vi "Teperature and FIeld Sweep_1022D.vi"() -> ()   [LabVIEW 2022 SP3]
uses:
  <vilib>/Analysis/baseanly.llb/Mean (DBL).vi
  <vilib>/Utility/file.llb/Write Delimited Spreadsheet (DBL).vi
  <vilib>/Analysis/NI_AALBase.lvlib
panel:
  out "Rh1 B/A v F":cluster{dbl[], dbl[]}(graph)
  in  "?":bool
  out "Temperature Status":i32(ring) items=["TemperatureUnknown"=0, "Stable"=1, "Tracking"=2, "Near"=5, "Chasing"=6, "Filling"=7, "Standby"=10, "Disabled"=13, "ImpedanceNotFunction"=14, "TempFailure"=15]
  out "Field Status":i32(ring) items=["MagnetUnknown"=0, "StablePersistent"=1, "WarmingSwitch"=2, "CoolingSwitch"=3, "StableDriven"=4, "Iterating"=5, "Charging"=6, "Discharging"=7, "CurrentError"=8, "MagnetFailure"=15]
  out "Field":dbl
  out "Temperature":dbl
  in  "Initialize":bool
  in  "System Stablization (s)":dbl=0.1 format="%#_13g"
  in  "Low Value (Oe)":dbl=-30000.0
  in  "High Value (Oe)":dbl=30000.0
  in  "Sweep Field Approach":i32(ring) items=["Linear", "NoOvershoot", "Oscillate"]
  in  "Sweep F Rate (Oe/s)":dbl=200.0 format="%#_13g"
  in  "Sweep F mode":i32(ring) items=["Persistent", "Driven"]
  in  "Set Fixed T":dbl=2.0
  in  "Fixed Temperature Approach":i32(ring)=1 items=["FastSettle", "NoOvershoot"]
  in  "FIxed T  Rate (K/min)":dbl=20.0
  out "PhaseA-F":cluster{dbl[], dbl[]}(graph)
  out "RA-F":cluster{dbl[], dbl[]}(graph)
  out "Phaseh1B-F":cluster{dbl[], dbl[]}(graph)
  out "Rh1B-F":cluster{dbl[], dbl[]}(graph)
  out "phase B 2":dbl
  in  "Phase B 2":u16(ring)=3 items=["X", "Y", "R", "Theta", "Frequency", "Noise", "Xh1", "Yh1", "Rh1", "Theta h1", "Xh2", "Yh2", "Rh2", "Theta h2"]
  out "phase A 2":dbl
  in  "Phase A 2":u16(ring)=3 items=["X", "Y", "R", "Theta", "Frequency", "Noise", "Xh1", "Yh1", "Rh1", "Theta h1", "Xh2", "Yh2", "Rh2", "Theta h2"]
  out "para1 Measurement (mV) 2":dbl=1.49013e-07
  in  "F Clear Plot A":bool
  in  "Parameter A 2":u16(ring)=2 items=["X", "Y", "R", "Theta", "Frequency", "Noise", "Xh1", "Yh1", "Rh1", "Theta h1", "Xh2", "Yh2", "Rh2", "Theta h2"]
  out "para2 Measurement (uV) 2":dbl=1.49013e-07
  in  "F Clear Plot B":bool
  in  "Parameter B 2":u16(ring)=2 items=["X", "Y", "R", "Theta", "Frequency", "Noise", "Xh1", "Yh1", "Rh1", "Theta h1", "Xh2", "Yh2", "Rh2", "Theta h2"]
  out "Field Setting":dbl format="%#_13g"
  out "Fixed Temperature":dbl
  out "Measured Field":dbl
  out "Field Status":i32(ring) items=["MagnetUnknown"=0, "StablePersistent"=1, "WarmingSwitch"=2, "CoolingSwitch"=3, "StableDriven"=4, "Iterating"=5, "Charging"=6, "Discharging"=7, "CurrentError"=8, "MagnetFailure"=15]
  out "Temperature Status":i32(ring) items=["TemperatureUnknown"=0, "Stable"=1, "Tracking"=2, "Near"=5, "Chasing"=6, "Filling"=7, "Standby"=10, "Disabled"=13, "ImpedanceNotFunction"=14, "TempFailure"=15]
  out "Measuring F":bool
  in  "Step(Oe)":i32=2000
  out "F loop run":i32
  out "Temperature Status":i32(ring) items=["TemperatureUnknown"=0, "Stable"=1, "Tracking"=2, "Near"=5, "Chasing"=6, "Filling"=7, "Standby"=10, "Disabled"=13, "ImpedanceNotFunction"=14, "TempFailure"=15]
  out "Field Status":i32(ring) items=["MagnetUnknown"=0, "StablePersistent"=1, "WarmingSwitch"=2, "CoolingSwitch"=3, "StableDriven"=4, "Iterating"=5, "Charging"=6, "Discharging"=7, "CurrentError"=8, "MagnetFailure"=15]
  out "Fixed Field":dbl
  out "Measured Temperature":dbl
  in  "Delay(T/F)":dbl=3000.0
  in  "Set FIxed F (Oe)":dbl format="%#_13g"
  in  "Fixed Field Approach":i32(ring) items=["Linear", "NoOvershoot", "Oscillate"]
  in  "FIxed F Rate (Oe/s)":dbl=100.0 format="%#_13g"
  in  "Fixed F mode":i32(ring) items=["Persistent", "Driven"]
  in  "Sweep Temperature Approach":i32(ring)=1 items=["FastSettle", "NoOvershoot"]
  in  "Sweep T  Rate (K/min)":dbl=10.0
  in  "Sweep T/F":bool
  in  "Remote":bool=TRUE
  in  "IP Address":string="169.254.170.239"
  out "Measuring T":bool
  in  "A Sine Output Amplitude (V)":sgl=0.1
  in  "path (folder + filename)":string="G:\\My Drive\\Opticool\\Measurement\\TF dependence\\TaI21_A1615_B166_267Hz_20kOhm"
  in  "LOCKIN address":refnum<visa-resource-name>="COM3"
  out "PhaseA-T":cluster{dbl[], dbl[]}(graph)
  out "RA-T":cluster{dbl[], dbl[]}(graph)
  out "Phaseh1-T":cluster{dbl[], dbl[]}(graph)
  out "Rh1B-T":cluster{dbl[], dbl[]}(graph)
  out "phase B":dbl
  in  "Phase B":u16(ring)=9 items=["X", "Y", "R", "Theta", "Frequency", "Noise", "Xh1", "Yh1", "Rh1", "Theta h1", "Xh2", "Yh2", "Rh2", "Theta h2"]
  out "phase A":dbl
  in  "Phase A":u16(ring)=3 items=["X", "Y", "R", "Theta", "Frequency", "Noise", "Xh1", "Yh1", "Rh1", "Theta h1", "Xh2", "Yh2", "Rh2", "Theta h2"]
  out "para1 Measurement (mV)":dbl=1.49013e-07
  in  "T Clear Plot A":bool
  in  "Parameter A":u16(ring)=2 items=["X", "Y", "R", "Theta", "Frequency", "Noise", "Xh1", "Yh1", "Rh1", "Theta h1", "Xh2", "Yh2", "Rh2", "Theta h2"]
  out "para2 Measurement (uV)":dbl=1.49013e-07
  in  "T Clear Plot B":bool
  in  "Parameter B":u16(ring)=8 items=["X", "Y", "R", "Theta", "Frequency", "Noise", "Xh1", "Yh1", "Rh1", "Theta h1", "Xh2", "Yh2", "Rh2", "Theta h2"]
  out "Temperature Setting":dbl format="%#_13g"
  in  "Save data or not":bool=TRUE
  in  "Step(K)":i32=10
  out "T loop run":i32
  in  "B frequency":dbl=267.7 format="%#_13g"
  in  "B Input Connection (0: Single-Ended)":u16(ring)=1 items=["Single-Ended Voltage", "Differential Voltage", "1 MOhm Current Gain", "100 MOhm Current Gain"]
  in  "B harmonic 1":u8=2
  in  "B harmonic 2":u8=3
  in  "B reference Manual Phase":dbl=-59.75
  in  "auto phase B":bool=TRUE
  in  "B Sample time (s)":dbl=0.001 min=0.001 max=100.0 step=0.001
  in  "B Sensitivity":u16(ring)=20 items=["1 nV/fA", "2 nV/fA", "5 nV/fA", "10 nV/fA", "20 nV/fA", "50 nV/fA", "100 nV/fA", "200 nV/fA", "500 nV/fA", "1 uV/pA", "2 uV/pA", "5 uV/pA", "10 uV/pA", "20 uV/pA", "50 uV/pA", "100 uV/pA", "200 uV/pA", "500 uV/pA", "1 mV/nA", "2 mV/nA", "5 mV/nA", "10 mV/nA", "20 mV/nA", "50 mV/nA", "100 mV/nA", "200 mV/nA", "500 mV/nA", "1 V/uA"]
  in  "Enable Sync Filter B (open when f<200Hz)":bool
  in  "B Time Constant":u8(ring)=9 items=["10 us", "30 us", "100 us", "300 us", "1 ms", "3 ms", "10 ms", "30 ms", "100 ms", "300 ms", "1 s", "3 s", "10 s", "30 s", "100 s", "300 s", "1 ks", "3 ks"]
  in  "B Reference Source":u8(ring) items=["External", "Internal", "Internal Sweep", "Channel-A"]
  in  "B Low Pass Filter Slope":u8(ring)=2 items=["6 dB/oct", "12 dB/oct", "18 db/oct", "24 dB/oct"]
  in  "A frequency":dbl=267.7 format="%#_13g"
  in  "A Input Connection (0: Single-Ended)":u16(ring)=1 items=["Single-Ended Voltage", "Differential Voltage", "1 MOhm Current Gain", "100 MOhm Current Gain"]
  in  "A harmonic 1":u8=2
  in  "A harmonic 2":u8=3
  in  "A reference Manual Phase":dbl=-59.75
  in  "auto phase A":bool=TRUE
  in  "A Reference Source":u8(ring)=1 items=["External", "Internal", "Internal Sweep"]
  in  "A Sample time (s)":dbl=0.001 min=0.001 max=100.0 step=0.001
  in  "A Time Constant":u8(ring)=9 items=["10 us", "30 us", "100 us", "300 us", "1 ms", "3 ms", "10 ms", "30 ms", "100 ms", "300 ms", "1 s", "3 s", "10 s", "30 s", "100 s", "300 s", "1 ks", "3 ks"]
  in  "Enable Sync Filter A (open when f<200Hz)":bool
  in  "A Sensitivity":u16(ring)=20 items=["1 nV/fA", "2 nV/fA", "5 nV/fA", "10 nV/fA", "20 nV/fA", "50 nV/fA", "100 nV/fA", "200 nV/fA", "500 nV/fA", "1 uV/pA", "2 uV/pA", "5 uV/pA", "10 uV/pA", "20 uV/pA", "50 uV/pA", "100 uV/pA", "200 uV/pA", "500 uV/pA", "1 mV/nA", "2 mV/nA", "5 mV/nA", "10 mV/nA", "20 mV/nA", "50 mV/nA", "100 mV/nA", "200 mV/nA", "500 mV/nA", "1 V/uA"]
  in  "A Low Pass Filter Slope":u8(ring)=2 items=["6 dB/oct", "12 dB/oct", "18 db/oct", "24 dB/oct"]
  in  "stabilization(S)":dbl=0.1 format="%#_13g"
  in  "High Value (K)":dbl=300.0
  in  "Low Value (K)":dbl=2.0
  in  "loop #":i32=1
  # "Statue"
  # "Lock-in Setting"
  # "Channel A"
  # "Channel B"
  # "Sweep F Mesurement"
  # "Temprature and Field Setting"
  # "Sweep T Mesurement"
  # "Sweep F"
  # "Sweep T"
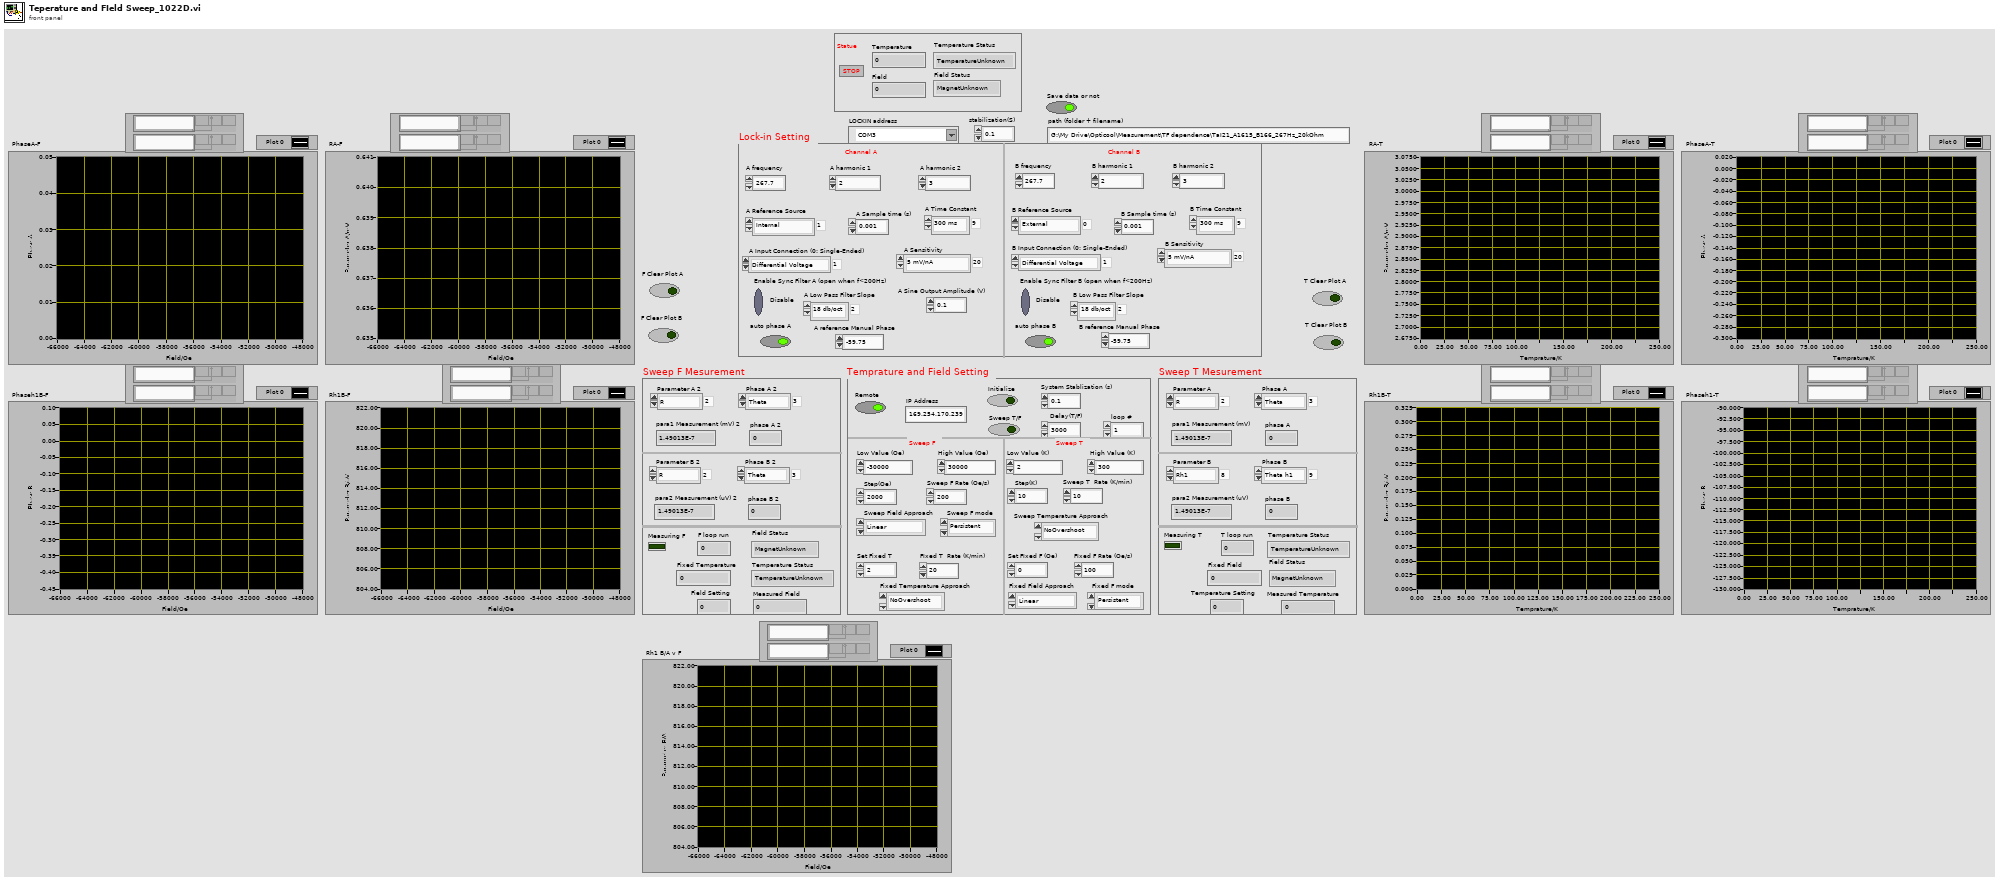
[diagram p1: front panel]
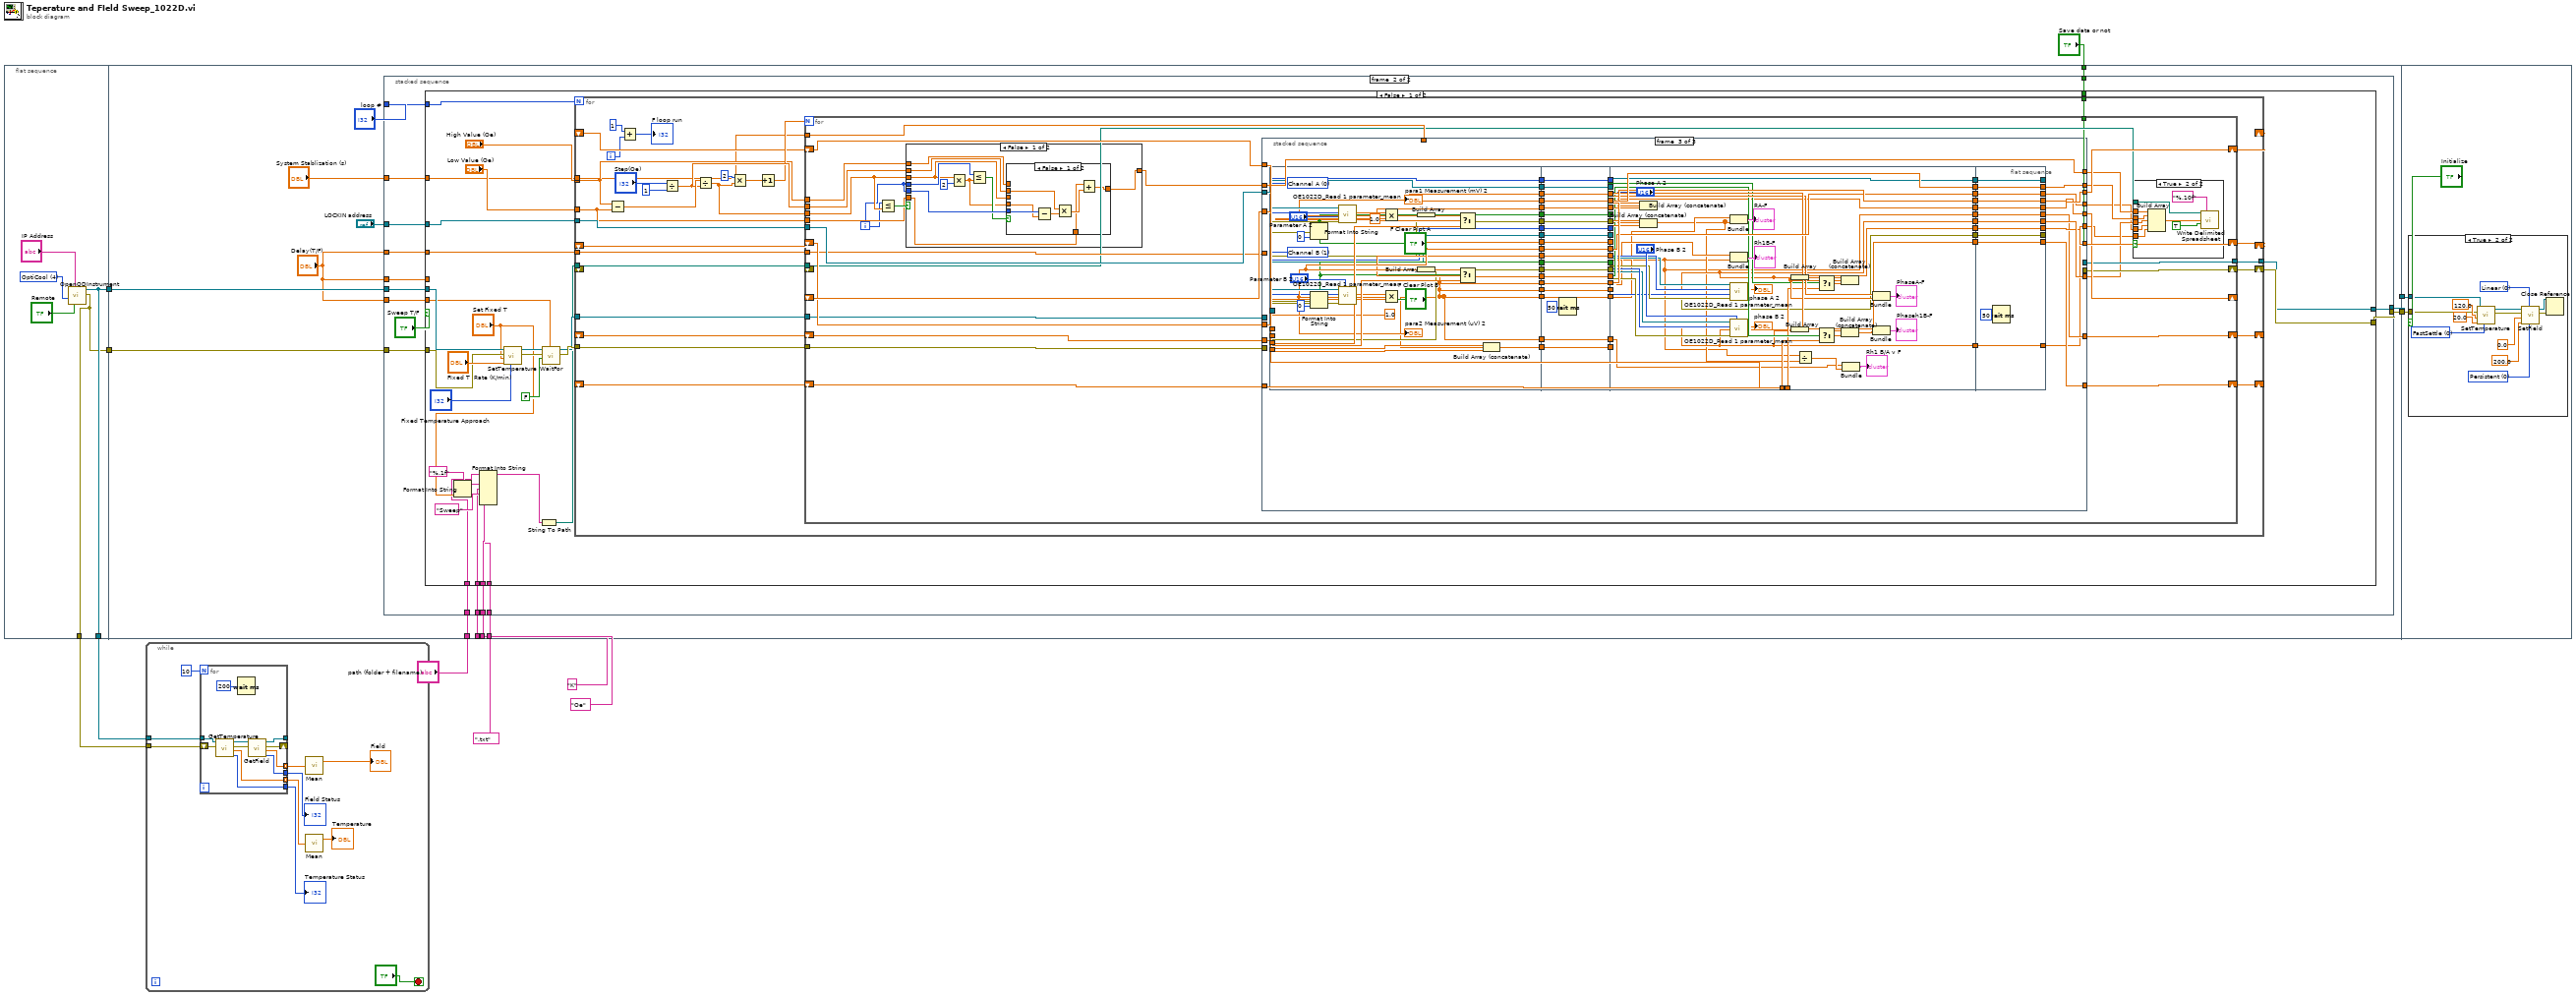
[diagram p0: block diagram]
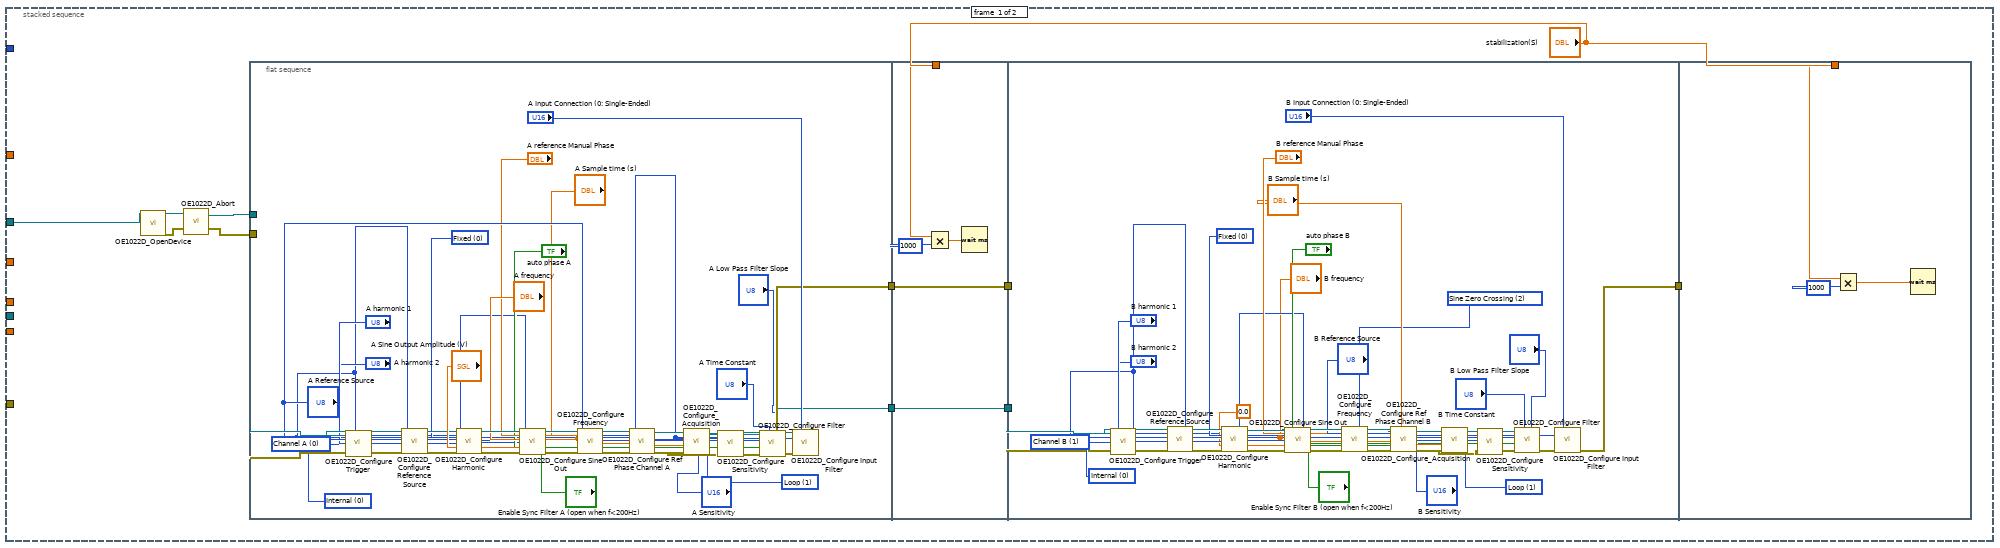
[diagram p2: hidden frame]
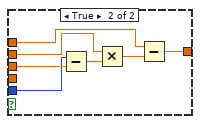
[diagram p4: hidden frame]
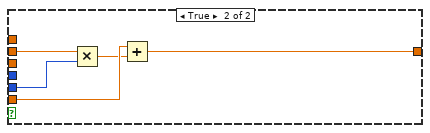
[diagram p5: hidden frame]
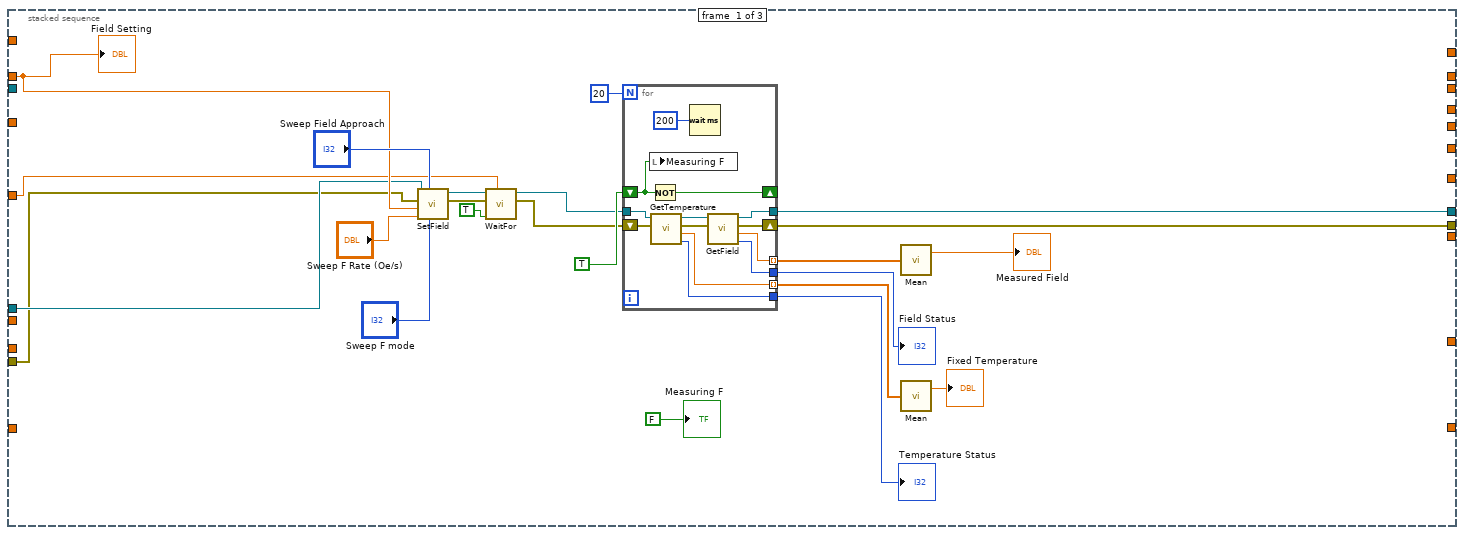
[diagram p6: hidden frame]
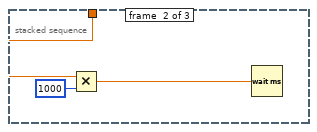
[diagram p7: hidden frame]
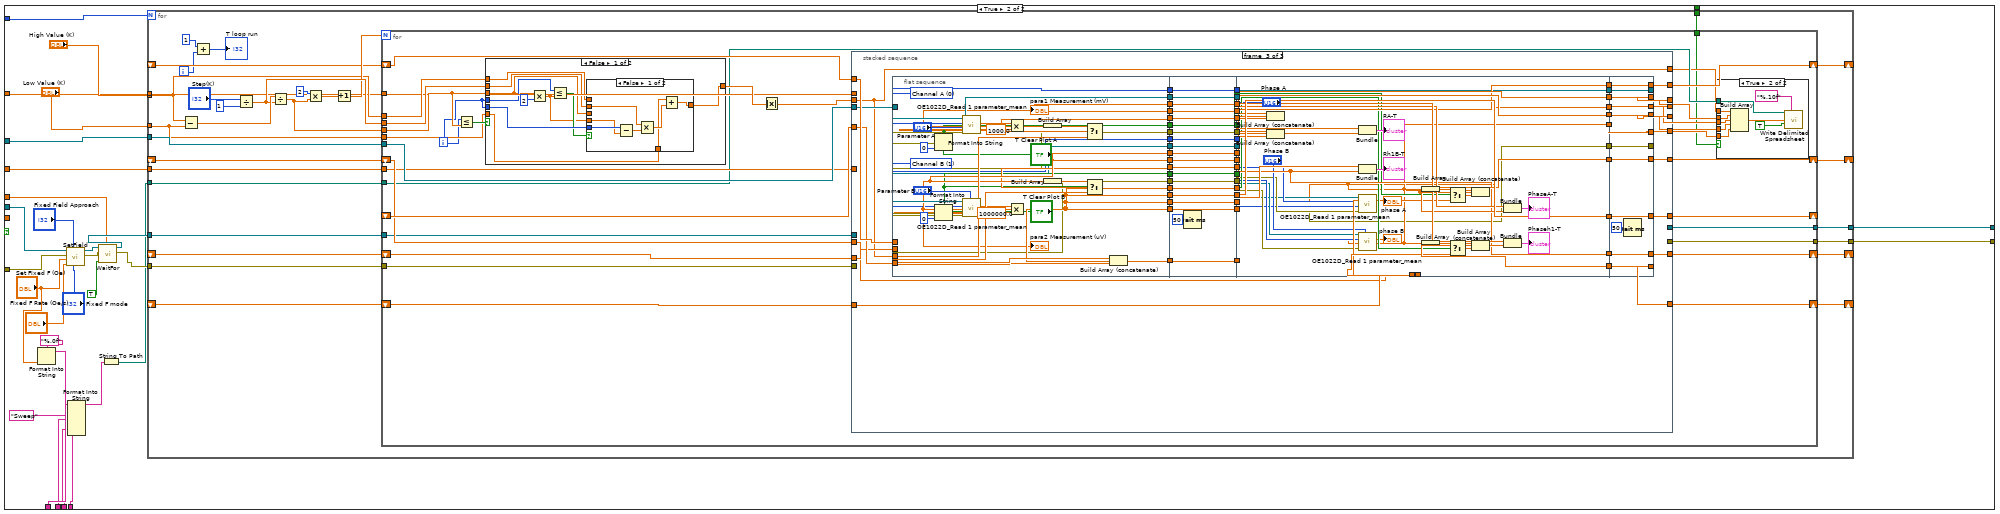
[diagram p8: hidden frame]
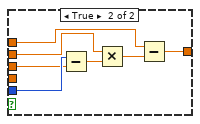
[diagram p10: hidden frame]
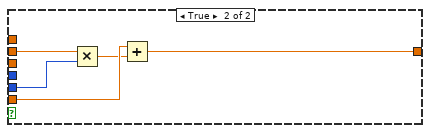
[diagram p11: hidden frame]
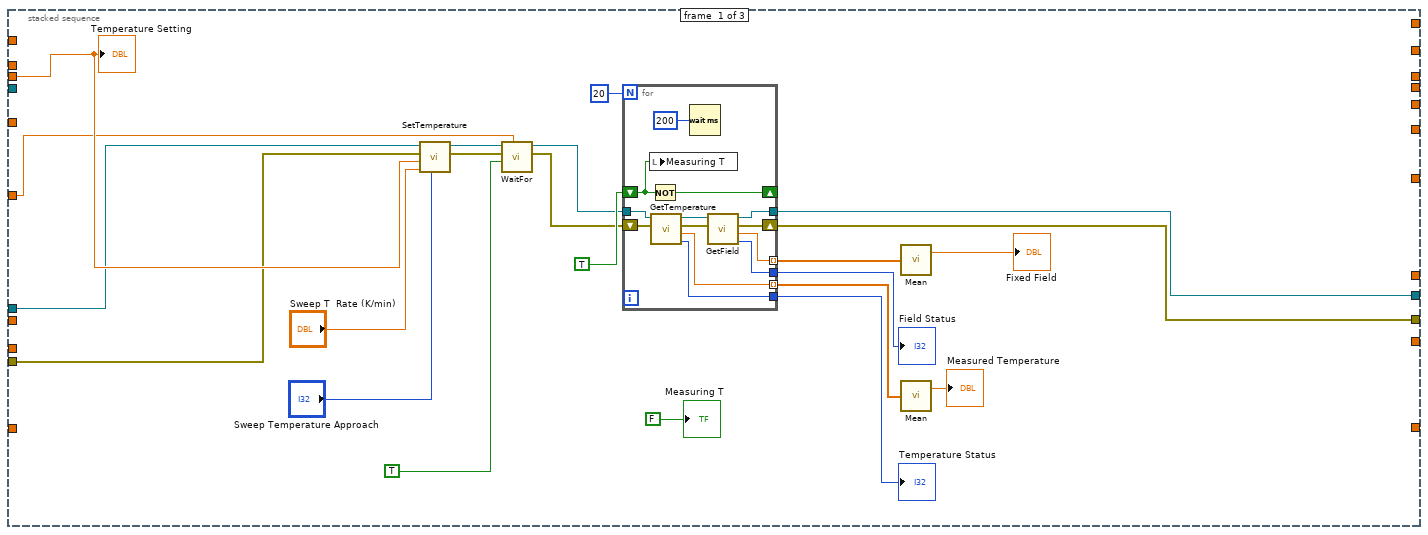
[diagram p12: hidden frame]
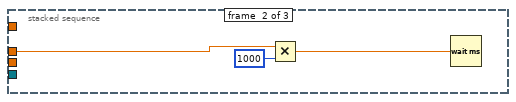
[diagram p13: hidden frame]
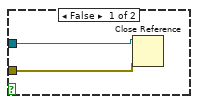
[diagram p14: hidden frame]
diagram:
  n1 = flat-sequence {
    tunnel: [w13] -> w11
    tunnel: [w12] -> w10
    tunnel: [w13] -> w3
    tunnel: [w12] -> w2
    tunnel: w11 -> [w27]
    tunnel: w10 -> [w26]
    tunnel: "path (folder + filename)" -> [w24]
    tunnel: "Oe" -> [w23]
    tunnel: "K" -> [w22]
    tunnel: ".txt" -> [w21]
    tunnel: [w19] -> w5
    tunnel: [w18] -> w4
    tunnel: "Save data or not" -> [w17]
    tunnel: w5 -> [w815]
    tunnel: w4 -> [w814]
    frame #0 {
      w14 = 4 items=["PPMS", "VersaLab", "DynaCool", "SVSM", "OptiCool"] ("InstrumentType")
      n2 = call "OpenQDInstrument.vi"("Remote"="Remote", "IP Address"="IP Address", "InstrumentType"=w14) -> ("error out"=w12:errorcluster, "Instrument Ref"=w13:refnum<k24>)  [unwired: 5 in]
    }
    frame #1 {
      n3 = stacked-sequence {
        tunnel: "LOCKIN address" -> [w32 w141]
        tunnel: "loop #" -> [_ w140]
        tunnel: w27 -> [_ w138]
        tunnel: w26 -> [_ w137]
        tunnel: "Delay(T/F)" -> [_ w136]
        tunnel: "Delay(T/F)" -> [_ w135]
        tunnel: "Delay(T/F)" -> [_ w134]
        tunnel: w24 -> [_ w133]
        tunnel: w23 -> [_ w132]
        tunnel: w22 -> [_ w131]
        tunnel: w21 -> [_ w130]
        tunnel: "System Stablization (s)" -> [_ w129]
        tunnel: [_ w128] -> w19
        tunnel: [_ w127] -> w18
        tunnel: w17 -> [_ w126]
        frame #0 {
          n4 = call "OE1022D_OpenDevice.vi"("VISA resource name"=w32) -> ("VISA资源名称输出"=w31:refnum<visa-resource-name>, "错误输出"=w33:errorcluster)  [unwired: 17 in]
          n5 = call "OE1022D_Abort.vi"("error in (no error)"=w33, "VISA resource name"=w31) -> ("error out"=w38:errorcluster, "VISA resource name out"=w39:refnum<visa-resource-name>)
          n6 = flat-sequence {
            tunnel: w39 -> [w79]
            tunnel: [w67] -> w37
            tunnel: w38 -> [w78]
            tunnel: [w55] -> w35
            tunnel: w37 -> [w84]
            tunnel: [w84] -> w36
            tunnel: w35 -> [w83]
            tunnel: [w83] -> w34
            tunnel: "stabilization(S)" -> [w80]
            tunnel: w36 -> [w105]
            tunnel: [w104] -> w40
            tunnel: w34 -> [w103]
            tunnel: w40 -> [_]
            tunnel: "stabilization(S)" -> [w123]
            frame #0 {
              w41 = u8 1 items=["Single", "Loop"] ("Sample Mode (Single/Loop)")
              w54 = u8 0 items=["Fixed", "Linear", "Log"] ("SineOut Mode")
              w56 = u16 0 items=["Internal", "External"] ("Trigger Source (0: Internal)")
              w45 = u8 0 items=["Channel A", "Channel B"] ("OE1022D A/B")
              n7 = call "OE1022D_Configure Trigger.vi"("Trigger Source (0: Internal)"=w56, "error in (no error)   2"=w78, "OE1022D A/B"=w45, "VISA resource name   2"=w79) -> ("error out   2"=w72:errorcluster, "VISA resource name out   2"=w73:refnum<visa-resource-name>)
              n8 = call "OE1022D_Configure Reference Source.vi"("VISA resource name"=w73, "OE1022D A/B"=w45, "Reference Source"="A Reference Source", "error in (no error)"=w72) -> ("VISA resource name out"=w71:refnum<visa-resource-name>, "error out"=w69:errorcluster)  [unwired: 14 in]
              n9 = call "OE1022D_Configure Harmonic.vi"("VISA resource name"=w71, "OE1022D A/B"=w45, "Harmonic 1"="A harmonic 1", "Harmonic 2"="A harmonic 2", "error in (no error)"=w69) -> ("VISA resource name out"=w70:refnum<visa-resource-name>, "error out"=w68:errorcluster)  [unwired: 13 in]
              n10 = call "OE1022D_Configure Sine Out.vi"("VISA resource name"=w70, "SineOut Mode"=w54, "OE1022D A/B"=w45, "Sine Output Amplitude (V)"="A Sine Output Amplitude (V)", "error in (no error)"=w68) -> ("VISA resource name out"=w76:refnum<visa-resource-name>, "error out"=w75:errorcluster)  [unwired: 9 in]
              n11 = call "OE1022D_Configure Frequency.vi"("VISA resource name"=w76, "OE1022D A/B"=w45, "Internal Frequency(Hz)"="A frequency", "error in (no error)"=w75) -> ("VISA resource name out"=w66:refnum<visa-resource-name>, "error out"=w63:errorcluster)  [unwired: 14 in]
              n12 = call "OE1022D_Configure Ref Phase Channel A.vi"("VISA resource name"=w66, "Reference Source"="A Reference Source", "Internal Frequency(Hz)"="A frequency", "Auto Phase (T: Enabled)"="auto phase A", "error in (no error)"=w63, "Manual Phase  (degree)"="A reference Manual Phase") -> ("VISA resource name out"=w65:refnum<visa-resource-name>, "error out"=w64:errorcluster)  [unwired: 12 in]
              n13 = call "OE1022D_Configure_Acquisition.vi"("VISA resource name"=w65, "OE1022D A/B"=w45, "Sample time (s)"="A Sample time (s)", "error in (no error)"=w64, "Sample Mode (Single/Loop)"=w41) -> ("VISA resource name out"=w48:refnum<visa-resource-name>, "error out"=w47:errorcluster)  [unwired: 3 in]
              n14 = call "OE1022D_Configure Sensitivity.vi"("VISA resource name"=w48, "OE1022D A/B"=w45, "Sensitivity"="A Sensitivity", "error in (no error)"=w47) -> ("VISA resource name out"=w52:refnum<visa-resource-name>, "error out"=w51:errorcluster)  [unwired: 14 in]
              n15 = call "OE1022D_Configure Filter.vi"("Low Pass Filter Slope (1: 12dB/oct)"="A Low Pass Filter Slope", "Time Constant (8: 100ms)"="A Time Constant", "error in (no error)"=w51, "Enable Sync Filter (F: Disable)"="Enable Sync Filter A (open when f<200Hz)", "OE1022D A/B"=w45, "VISA resource name"=w52) -> ("error out"=w49:errorcluster, "VISA resource name out"=w50:refnum<visa-resource-name>)  [unwired: 4 in]
              n16 = call "OE1022D_Configure Input Filter.vi"("VISA resource name"=w50, "Input Source"="A Input Connection (0: Single-Ended)", "OE1022D A/B"=w45, "error in (no error)"=w49) -> ("VISA resource name out"=w55:refnum<visa-resource-name>, "error out"=w67:errorcluster)  [unwired: 10 in]
            }
            frame #1 {
              n17 = Multiply(x=w80, y=1000) -> (x*y=w82:dbl)
              n18 = Wait (ms)(milliseconds to wait=w82) -> ()  [unwired: 1 out]
            }
            frame #2 {
              w85 = u8 1 items=["Single", "Loop"] ("Sample Mode (Single/Loop)")
              w87 = u8 2 items=["TTL Pos", "TTL Neg", "Sine Zero Crossing"] ("External Ref Trigger")
              w100 = u8 0 items=["Fixed", "Linear", "Log"] ("SineOut Mode")
              w106 = u16 0 items=["Internal", "External"] ("Trigger Source (0: Internal)")
              w92 = u8 1 items=["Channel A", "Channel B"] ("OE1022D A/B")
              n19 = call "OE1022D_Configure Trigger.vi"("Trigger Source (0: Internal)"=w106, "error in (no error)   2"=w105, "OE1022D A/B"=w92, "VISA resource name   2"=w103) -> ("error out   2"=w118:errorcluster, "VISA resource name out   2"=w119:refnum<visa-resource-name>)
              n20 = call "OE1022D_Configure Reference Source.vi"("VISA resource name"=w119, "OE1022D A/B"=w92, "error in (no error)"=w118) -> ("VISA resource name out"=w117:refnum<visa-resource-name>, "error out"=w115:errorcluster)  [unwired: 15 in]
              n21 = call "OE1022D_Configure Harmonic.vi"("VISA resource name"=w117, "OE1022D A/B"=w92, "Harmonic 1"="B harmonic 1", "Harmonic 2"="B harmonic 2", "error in (no error)"=w115) -> ("VISA resource name out"=w116:refnum<visa-resource-name>, "error out"=w114:errorcluster)  [unwired: 13 in]
              n22 = call "OE1022D_Configure Sine Out.vi"("VISA resource name"=w116, "SineOut Mode"=w100, "OE1022D A/B"=w92, "Sine Output Amplitude (V)"=sgl 0.0, "error in (no error)"=w114) -> ("VISA resource name out"=w121:refnum<visa-resource-name>, "error out"=w120:errorcluster)  [unwired: 9 in]
              n23 = call "OE1022D_Configure Frequency.vi"("VISA resource name"=w121, "OE1022D A/B"=w92, "Internal Frequency(Hz)"="B frequency", "error in (no error)"=w120) -> ("VISA resource name out"=w113:refnum<visa-resource-name>, "error out"=w110:errorcluster)  [unwired: 14 in]
              n24 = call "OE1022D_Configure Ref Phase Channel B.vi"("VISA resource name"=w113, "Reference Source"="B Reference Source", "External Ref Trigger"=w87, "Internal Frequency(Hz)"="B frequency", "Auto Phase (T: Enabled)"="auto phase B", "error in (no error)"=w110, "Manual Phase  (degree)"="B reference Manual Phase") -> ("VISA resource name out"=w112:refnum<visa-resource-name>, "error out"=w111:errorcluster)  [unwired: 11 in]
              n25 = call "OE1022D_Configure_Acquisition.vi"("VISA resource name"=w112, "OE1022D A/B"=w92, "Sample time (s)"="B Sample time (s)", "error in (no error)"=w111, "Sample Mode (Single/Loop)"=w85) -> ("VISA resource name out"=w93:refnum<visa-resource-name>, "error out"=w94:errorcluster)  [unwired: 3 in]
              n26 = call "OE1022D_Configure Sensitivity.vi"("VISA resource name"=w93, "OE1022D A/B"=w92, "Sensitivity"="B Sensitivity", "error in (no error)"=w94) -> ("VISA resource name out"=w97:refnum<visa-resource-name>, "error out"=w96:errorcluster)  [unwired: 14 in]
              n27 = call "OE1022D_Configure Filter.vi"("Low Pass Filter Slope (1: 12dB/oct)"="B Low Pass Filter Slope", "Time Constant (8: 100ms)"="B Time Constant", "error in (no error)"=w96, "Enable Sync Filter (F: Disable)"="Enable Sync Filter B (open when f<200Hz)", "OE1022D A/B"=w92, "VISA resource name"=w97) -> ("error out"=w95:errorcluster)  [unwired: 4 in, 1 out]
              n28 = call "OE1022D_Configure Input Filter.vi"("Input Source"="B Input Connection (0: Single-Ended)", "OE1022D A/B"=w92, "error in (no error)"=w95) -> ("error out"=w104:errorcluster)  [unwired: 11 in, 1 out]
            }
            frame #3 {
              n29 = Multiply(x=w123, y=1000) -> (x*y=w125:dbl)
              n30 = Wait (ms)(milliseconds to wait=w125) -> ()  [unwired: 1 out]
            }
          }
        }
        frame #1 {
          n31 = case shown="False" "Sweep T/F" {
            tunnel: w141 -> [w169 w509]
            tunnel: w140 -> [w170 w508]
            tunnel: w138 -> [w161 w504]
            tunnel: w137 -> [w162 w503]
            tunnel: w136 -> [_ w497]
            tunnel: w135 -> [w168 w496]
            tunnel: w134 -> [w160 _]
            tunnel: w133 -> [w151 w491]
            tunnel: w132 -> [w150 w487]
            tunnel: w131 -> [w149 w488]
            tunnel: w130 -> [w148 w486]
            tunnel: w129 -> [w145 w483]
            tunnel: [w144 w482] -> w128
            tunnel: [w143 w481] -> w127
            tunnel: w126 -> [w142 w480]
            frame False {
              n32 = Format Into String(format string="%.1f", "Set Fixed T") -> (resulting string=w154:string)  [unwired: 2 in, 1 out]
              n33 = Format Into String(initial string=w151, w154, w149, "Sweep", w150, w148) -> (resulting string=w155:string)  [unwired: 2 in, 1 out]
              n34 = call "SetTemperature.vi"("Approach"="Fixed Temperature Approach", "Rate"="FIxed T  Rate (K/min)", "Temperature"="Set Fixed T", "error in (no error)"=w162, "Instrument Ref In"=w161) -> ("error out"=w163:errorcluster, "Instrument Ref Out"=w164:refnum<k24>)  [unwired: 2 in, 1 out]
              n35 = String To Path(string=w155) -> (path=w152:path)
              n36 = call "WaitFor.vi"("Delay"=w160, "Wait For Temperature"=FALSE ("WaitForTemperature"), "error in (no error)"=w163, "Instrument Ref In"=w164) -> ("error out"=w159:errorcluster, "Instrument Ref Out"=w158:refnum<k24>)  [unwired: 6 in]
              n37 = for {
                N: w170 -> [_]
                tunnel: w169 -> [w200]
                tunnel: "Low Value (Oe)" -> [w194]
                tunnel: "High Value (Oe)" -> [w184]
                tunnel: w152 -> [w193]
                shift-right: [w189] -> _
                shift-left: _ -> [w188]
                shift-right: [w183] -> _
                shift-left: _ -> [w182]
                shift-right: [w181] -> _
                shift-left: _ -> [w180]
                shift-right: [w179] -> _
                shift-left: _ -> [w178]
                tunnel: w158 -> [w177]
                tunnel: w159 -> [w176]
                tunnel: w168 -> [w175]
                tunnel: w145 -> [w174]
                shift-right: [w173] -> w144
                shift-left: _ -> [_]
                tunnel: [w172] -> w143
                tunnel: w142 -> [w171]
                i -> [w186]
                n38 = Subtract(x=w184, y=w194) -> (x-y=w196:dbl)
                n39 = Add(x=1, y=w186) -> (x+y=→"F loop run":i32)
                n40 = Divide(x="Step(Oe)", y=1) -> (x/y=w195:dbl)
                n41 = Divide(x=w196, y=w195) -> (x/y=w192:dbl)
                n42 = Multiply(x=2, y=w192) -> (x*y=w191:dbl)
                n43 = Increment(x=w191) -> (x+1=w190:dbl)
                n44 = for {
                  N: w190 -> [_]
                  tunnel: w200 -> [w231]
                  tunnel: w195 -> [w227]
                  shift-right: [w219] -> w189
                  shift-left: w188 -> [w230]
                  tunnel: w192 -> [w225]
                  tunnel: w194 -> [w228]
                  tunnel: w184 -> [w226]
                  tunnel: w193 -> [w207]
                  shift-right: [w218] -> _
                  shift-left: _ -> [w222]
                  shift-right: [w221] -> w183
                  shift-left: w182 -> [w220]
                  shift-right: [w217] -> w181
                  shift-left: w180 -> [w216]
                  shift-right: [w215] -> w179
                  shift-left: w178 -> [w214]
                  tunnel: w177 -> [w213]
                  tunnel: w176 -> [w212]
                  tunnel: w175 -> [w211]
                  tunnel: w174 -> [w210]
                  shift-right: [w209] -> w173
                  shift-left: _ -> [_]
                  tunnel: [w208] -> w172
                  tunnel: w171 -> [w201]
                  i -> [w224]
                  n45 = Less Or Equal?(x=w224, y=w225) -> (x <= y?=w229:bool)
                  n46 = case shown="False" w229 {
                    tunnel: w228 -> [w241 w269]
                    tunnel: w224 -> [w250 w268]
                    tunnel: w227 -> [w249 w267]
                    tunnel: [w247 w265] -> w223
                    tunnel: w226 -> [w248 _]
                    tunnel: w225 -> [w243 _]
                    tunnel: w224 -> [w246 _]
                    frame False {
                      n47 = Multiply(x=w243, y=2) -> (x*y=w242:dbl)
                      n48 = Less Or Equal?(x=w246, y=w242) -> (x <= y?=w244:bool)
                      n49 = case shown="False" w244 {
                        tunnel: w250 -> [w257 w264]
                        tunnel: w249 -> [w255 w262]
                        tunnel: w248 -> [_ w260]
                        tunnel: [w253 w259] -> w247
                        tunnel: w243 -> [_ w258]
                        tunnel: w242 -> [w252 _]
                        tunnel: w241 -> [w251 _]
                        frame False {
                          n50 = Subtract(x=w257, y=w252) -> (x-y=w256:dbl)
                          n51 = Multiply(x=w255, y=w256) -> (x*y=w254:dbl)
                          n52 = Add(x=w251, y=w254) -> (x+y=w253:dbl)
                        }
                        frame True {
                          n53 = Subtract(x=w264, y=w258) -> (x-y=w263:dbl)
                          n54 = Multiply(x=w262, y=w263) -> (x*y=w261:dbl)
                          n55 = Subtract(x=w260, y=w261) -> (x-y=w259:dbl)
                        }
                      }
                    }
                    frame True {
                      n56 = Multiply(x=w267, y=w268) -> (x*y=w266:dbl)
                      n57 = Add(x=w269, y=w266) -> (x+y=w265:dbl)
                    }
                  }
                  n58 = stacked-sequence {
                    tunnel: w231 -> [_ _ w373]
                    tunnel: w223 -> [w275 _ w372]
                    tunnel: w230 -> [_ _ w375]
                    tunnel: [_ _ w374] -> w219
                    tunnel: [_ _ w311] -> w205
                    tunnel: [_ _ w372] -> w206
                    tunnel: [_ _ w371] -> w218
                    tunnel: w222 -> [_ _ w370]
                    tunnel: [_ _ w369] -> w204
                    tunnel: [_ _ w368] -> w221
                    tunnel: w220 -> [_ _ w361]
                    tunnel: [_ _ w367] -> w217
                    tunnel: w216 -> [_ _ w362]
                    tunnel: [_ _ w366] -> w215
                    tunnel: w214 -> [_ _ w365]
                    tunnel: [_ _ w364] -> w202
                    tunnel: [_ _ w363] -> w203
                    tunnel: w213 -> [w274 _ _]
                    tunnel: w212 -> [w273 _ _]
                    tunnel: w211 -> [w272 _ _]
                    tunnel: w210 -> [_ w306 _]
                    tunnel: [w271 _ _] -> w209
                    tunnel: [w270 _ _] -> w208
                    frame #0 {
                      n59 = call "SetField.vi"("Mode"="Sweep F mode", "Approach"="Sweep Field Approach", "Rate"="Sweep F Rate (Oe/s)", "Field"=w275, "error in (no error)"=w273, "Instrument Ref In"=w274) -> ("error out"=w279:errorcluster, "Instrument Ref Out"=w280:refnum<k24>)  [unwired: 1 in, 1 out]
                      n60 = call "WaitFor.vi"("Delay"=w272, "Wait For Field"=TRUE, "error in (no error)"=w279, "Instrument Ref In"=w280) -> ("error out"=w277:errorcluster, "Instrument Ref Out"=w276:refnum<k24>)  [unwired: 6 in]
                      n61 = for {
                        N: 20 -> [_]
                        shift-right: [w305] -> _
                        shift-left: TRUE -> [w303]
                        shift-right: [w300] -> w271
                        shift-left: w277 -> [w302]
                        tunnel: w276 -> [w299]
                        tunnel: [w297] -> w270
                        tunnel: [w294] -> w290
                        tunnel: [w293] -> w289
                        tunnel: [w295] -> w287 mode=indexing
                        tunnel: [w296] -> w288 mode=indexing
                        n62 = local write "Measuring F"(w303) -> ()
                        n63 = Not(x=w303) -> (.not. x?=w305:bool)
                        n64 = call "GetTemperature.vi"("error in (no error)"=w302, "Instrument Ref In"=w299) -> ("Temperature\nStatus"=w293:i32, "Temperature"=w296:dbl, "error out"=w301:errorcluster, "Instrument Ref Out"=w298:refnum<k24>)  [unwired: 3 in, 1 out]
                        n65 = Wait (ms)(milliseconds to wait=u32 200) -> ()  [unwired: 1 out]
                        n66 = call "GetField.vi"("error in (no error)"=w301, "Instrument Ref In"=w298) -> ("Field\nStatus"=w294:i32, "Field"=w295:dbl, "error out"=w300:errorcluster, "Instrument Ref Out"=w297:refnum<k24>)  [unwired: 3 in, 1 out]
                      }
                      "Field Status" <- w290
                      "Temperature Status" <- w289
                      n67 = call-poly <vilib>:"Mean.vi"("X"=w287) -> ("mean"=→"Measured Field":dbl)  [unwired: 1 out]
                      n68 = call-poly <vilib>:"Mean.vi"("X"=w288) -> ("mean"=→"Fixed Temperature":dbl)  [unwired: 1 out]
                      "Field Setting" <- w275
                      "Measuring F" <- FALSE
                    }
                    frame #1 {
                      n69 = Multiply(x=w306, y=1000) -> (x*y=w308:dbl)
                      n70 = Wait (ms)(milliseconds to wait=w308) -> ()  [unwired: 1 out]
                    }
                    frame #2 {
                      n71 = flat-sequence {
                        tunnel: w375 -> [w403]
                        tunnel: w373 -> [w394]
                        tunnel: w372 -> [w402]
                        tunnel: w370 -> [w401]
                        tunnel: w365 -> [w392]
                        tunnel: [w399] -> w360
                        tunnel: [w387] -> w358
                        tunnel: [w376] -> w356
                        tunnel: [w385] -> w354
                        tunnel: [w376] -> w352
                        tunnel: [w376] -> w350
                        tunnel: [w376] -> w348
                        tunnel: [w376] -> w346
                        tunnel: [w387] -> w344
                        tunnel: [w386] -> w342
                        tunnel: [w385] -> w340
                        tunnel: [w384] -> w338
                        tunnel: ["F Clear Plot B"] -> w336
                        tunnel: ["F Clear Plot A"] -> w334
                        tunnel: [w381] -> w332
                        tunnel: [w380] -> w330
                        tunnel: [w379] -> w328
                        tunnel: [w378] -> w326
                        tunnel: [w377] -> w324
                        tunnel: [w376] -> w309
                        tunnel: w360 -> [w426]
                        tunnel: [w426] -> w359
                        tunnel: w358 -> [w425]
                        tunnel: [w425] -> w357
                        tunnel: w356 -> [w424]
                        tunnel: [w424] -> w355
                        tunnel: w354 -> [w423]
                        tunnel: [w423] -> w353
                        tunnel: w352 -> [w422]
                        tunnel: [w422] -> w351
                        tunnel: w350 -> [w421]
                        tunnel: [w421] -> w349
                        tunnel: w348 -> [w420]
                        tunnel: [w420] -> w347
                        tunnel: w346 -> [w419]
                        tunnel: [w419] -> w345
                        tunnel: w344 -> [w418]
                        tunnel: [w418] -> w343
                        tunnel: w342 -> [w417]
                        tunnel: [w417] -> w341
                        tunnel: w340 -> [w416]
                        tunnel: [w416] -> w339
                        tunnel: w338 -> [w415]
                        tunnel: [w415] -> w337
                        tunnel: w336 -> [w414]
                        tunnel: [w414] -> w335
                        tunnel: w334 -> [w413]
                        tunnel: [w413] -> w333
                        tunnel: w332 -> [w412]
                        tunnel: [w412] -> w331
                        tunnel: w330 -> [w411]
                        tunnel: [w411] -> w329
                        tunnel: w328 -> [w410]
                        tunnel: [w410] -> w327
                        tunnel: w326 -> [w409]
                        tunnel: [w409] -> w325
                        tunnel: w324 -> [w408]
                        tunnel: [w408] -> w323
                        tunnel: [w406] -> w310
                        tunnel: w309 -> [w406]
                        tunnel: w359 -> [w437]
                        tunnel: w357 -> [w467]
                        tunnel: w355 -> [w466]
                        tunnel: w353 -> [w465]
                        tunnel: w351 -> [w464]
                        tunnel: w349 -> [w433]
                        tunnel: w347 -> [w432]
                        tunnel: w345 -> [w460]
                        tunnel: w343 -> [w457]
                        tunnel: w341 -> [w456]
                        tunnel: w339 -> [w454]
                        tunnel: w337 -> [w453]
                        tunnel: w362 -> [w452]
                        tunnel: w335 -> [w451]
                        tunnel: w361 -> [w449]
                        tunnel: w333 -> [w448]
                        tunnel: w331 -> [w444]
                        tunnel: w329 -> [w443]
                        tunnel: w327 -> [w442]
                        tunnel: w325 -> [w439]
                        tunnel: w323 -> [w438]
                        tunnel: [w437] -> w322
                        tunnel: [w431] -> w321
                        tunnel: [w467] -> w320
                        tunnel: [w466] -> w319
                        tunnel: [w435] -> w318
                        tunnel: [w436] -> w317
                        tunnel: [w458] -> w316
                        tunnel: [w455] -> w315
                        tunnel: [w430] -> w314
                        tunnel: [w465] -> w313
                        tunnel: [w441] -> w312
                        tunnel: w310 -> [w428]
                        tunnel: [w469] -> w363
                        tunnel: [w470] -> w364
                        tunnel: [w471] -> w366
                        tunnel: [w472] -> w367
                        tunnel: [w473] -> w368
                        tunnel: [w474] -> _
                        tunnel: [w475] -> w369
                        tunnel: [w476] -> w371
                        tunnel: [w477] -> w311
                        tunnel: [w478] -> w374
                        tunnel: [w479] -> _
                        tunnel: w322 -> [w479]
                        tunnel: w321 -> [w478]
                        tunnel: w320 -> [w477]
                        tunnel: w319 -> [w476]
                        tunnel: w318 -> [w475]
                        tunnel: w317 -> [w474]
                        tunnel: w316 -> [w473]
                        tunnel: w315 -> [w472]
                        tunnel: w314 -> [w471]
                        tunnel: w313 -> [w470]
                        tunnel: w312 -> [w469]
                        frame #0 {
                          w380 = u8 1 items=["Channel A", "Channel B"] ("Channel A/B for Parameter1")
                          w377 = u8 0 items=["Channel A", "Channel B"] ("Channel A/B for Parameter1")
                          n72 = Format Into String(0) -> (error out=w400:errorcluster)  [unwired: 3 in, 1 out]
                          n73 = Format Into String(0) -> (error out=w395:errorcluster)  [unwired: 3 in, 1 out]
                          n74 = call "OE1022D_Read 1 parameter_mean.vi"("错误输入（无错误）"=w400, "Parameter"="Parameter A 2", "Channel (0: A)"=w377, "VISA resource name"=w394) -> ("error out"=w378:errorcluster, "Measurement"=w389:dbl, "VISA resource name out"=w399:refnum<visa-resource-name>)  [unwired: 5 in]
                          n75 = call "OE1022D_Read 1 parameter_mean.vi"("Parameter 2"="Parameter B 2", "错误输入（无错误）"=w395, "Channel (0: A)"=w380, "VISA resource name"=w394) -> ("error out"=w381:errorcluster, "Measurement"=w388:dbl, "VISA resource name out"=w379:refnum<visa-resource-name>)  [unwired: 5 in]
                          n76 = Multiply(x=w389, y=1.0) -> (x*y=w387:dbl)
                          "para1 Measurement (mV) 2" <- w387
                          n77 = Multiply(x=w388, y=1.0) -> (x*y=w385:dbl)
                          "para2 Measurement (uV) 2" <- w385
                          n78 = Build Array(w387) -> (w404:dbl[])
                          n79 = Build Array(w385) -> (w396:dbl[])
                          n80 = Select(t=w404, s="F Clear Plot A", f=w403) -> (s? t:f=w386:dbl[])
                          n81 = Select(t=w396, s="F Clear Plot B", f=w392) -> (s? t:f=w384:dbl[])
                          n82 = Build Array (concatenate)(w402, w401) -> (w376:dbl[])
                        }
                        frame #1 {
                          n83 = Wait (ms)(milliseconds to wait=u32 50) -> ()  [unwired: 1 out]
                        }
                        frame #2 {
                          n84 = Build Array (concatenate)(w457, w456) -> (w431:dbl[])
                          n85 = Build Array (concatenate)(w454, w453) -> (w430:dbl[])
                          n86 = Bundle(w432, w431) -> (→"RA-F":cluster{dbl[], dbl[]})  [unwired: 1 in]
                          n87 = Bundle(w433, w430) -> (→"Rh1B-F":cluster{dbl[], dbl[]})  [unwired: 1 in]
                          n88 = call "OE1022D_Read 1 parameter_mean.vi"("错误输入（无错误）"=w439, "Parameter"="Phase A 2", "Channel (0: A)"=w438, "VISA resource name"=w437) -> ("error out"=w436:errorcluster, "Measurement"=w435:dbl)  [unwired: 5 in, 1 out]
                          "phase A 2" <- w435
                          n89 = call "OE1022D_Read 1 parameter_mean.vi"("Parameter 2"="Phase B 2", "错误输入（无错误）"=w444, "Channel (0: A)"=w443, "VISA resource name"=w442) -> ("Measurement"=w441:dbl)  [unwired: 5 in, 2 out]
                          "phase B 2" <- w441
                          n90 = Build Array(w435) -> (w445:dbl[])
                          n91 = Build Array(w441) -> (w446:dbl[])
                          n92 = Divide(x=w430, y=w431) -> (x/y=w429:dbl[])
                          n93 = Select(t=w445, s=w448, f=w449) -> (s? t:f=w447:dbl[])
                          n94 = Select(t=w446, s=w451, f=w452) -> (s? t:f=w450:dbl[])
                          n95 = Build Array (concatenate)(w435, w447) -> (w458:dbl[])
                          n96 = Build Array (concatenate)(w441, w450) -> (w455:dbl[])
                          n97 = Bundle(w428, w429) -> (→"Rh1 B/A v F":cluster{dbl[], dbl[]})  [unwired: 1 in]
                          n98 = Bundle(w460, w458) -> (→"PhaseA-F":cluster{dbl[], dbl[]})  [unwired: 1 in]
                          n99 = Bundle(w464, w455) -> (→"Phaseh1B-F":cluster{dbl[], dbl[]})  [unwired: 1 in]
                        }
                        frame #3 {
                          n100 = Wait (ms)(milliseconds to wait=u32 50) -> ()  [unwired: 1 out]
                        }
                      }
                    }
                  }
                  n101 = case shown="True" w201 {
                    tunnel: w205 -> [_ w235]
                    tunnel: w206 -> [_ w240]
                    tunnel: w207 -> [_ w238]
                    tunnel: w204 -> [_ w234]
                    tunnel: w202 -> [_ w233]
                    tunnel: w203 -> [_ w232]
                    frame False {
                    }
                    frame True {
                      n102 = Build Array(w240, w235, w234, w233, w232) -> (w237:dbl[])
                      n103 = call-poly <vilib>:"Write Delimited Spreadsheet.vi"("file path (dialog if empty)"=w238, "format (%.3f)"="%.10f", "1D data"=w237, "append to file? (new file:F)"=TRUE) -> ()  [unwired: 10 in, 2 out]
                    }
                  }
                }
              }
            }
            frame True {
              n104 = Format Into String(format string="%.0f", "Set FIxed F (Oe)") -> (resulting string=w490:string)  [unwired: 2 in, 1 out]
              n105 = call "SetField.vi"("Mode"="Fixed F mode", "Approach"="Fixed Field Approach", "Rate"="FIxed F Rate (Oe/s)", "Field"="Set FIxed F (Oe)", "error in (no error)"=w503, "Instrument Ref In"=w504) -> ("error out"=w499:errorcluster, "Instrument Ref Out"=w501:refnum<k24>)  [unwired: 1 in, 1 out]
              n106 = Format Into String(initial string=w491, "Sweep", w488, w490, w487, w486) -> (resulting string=w493:string)  [unwired: 2 in, 1 out]
              n107 = call "WaitFor.vi"("Delay"=w497, "Wait For Field"=TRUE, "error in (no error)"=w499, "Instrument Ref In"=w501) -> ("error out"=w500:errorcluster, "Instrument Ref Out"=w502:refnum<k24>)  [unwired: 6 in]
              n108 = String To Path(string=w493) -> (path=w492:path)
              n109 = for {
                N: w508 -> [_]
                tunnel: w509 -> [w539]
                tunnel: "Low Value (K)" -> [w533]
                tunnel: "High Value (K)" -> [w523]
                tunnel: w492 -> [w532]
                shift-right: [w528] -> _
                shift-left: _ -> [w527]
                shift-right: [w522] -> _
                shift-left: _ -> [w521]
                shift-right: [w520] -> _
                shift-left: _ -> [w519]
                shift-right: [w518] -> _
                shift-left: _ -> [w517]
                tunnel: w502 -> [w516]
                tunnel: w500 -> [w515]
                tunnel: w496 -> [w514]
                tunnel: w483 -> [w513]
                tunnel: [w512] -> w482
                tunnel: [w511] -> w481
                tunnel: w480 -> [w510]
                i -> [w525]
                n110 = Subtract(x=w523, y=w533) -> (x-y=w535:dbl)
                n111 = Add(x=1, y=w525) -> (x+y=→"T loop run":i32)
                n112 = Divide(x="Step(K)", y=1) -> (x/y=w534:dbl)
                n113 = Divide(x=w535, y=w534) -> (x/y=w531:dbl)
                n114 = Multiply(x=2, y=w531) -> (x*y=w530:dbl)
                n115 = Increment(x=w530) -> (x+1=w529:dbl)
                n116 = for {
                  N: w529 -> [_]
                  tunnel: w539 -> [w571]
                  tunnel: w534 -> [w567]
                  shift-right: [w558] -> w528
                  shift-left: w527 -> [w570]
                  tunnel: w531 -> [w565]
                  tunnel: w533 -> [w568]
                  tunnel: w523 -> [w566]
                  tunnel: w532 -> [w542]
                  shift-right: [w547] -> _
                  shift-left: _ -> [w561]
                  shift-right: [w560] -> w522
                  shift-left: w521 -> [w559]
                  shift-right: [w557] -> w520
                  shift-left: w519 -> [w556]
                  shift-right: [w555] -> w518
                  shift-left: w517 -> [w554]
                  tunnel: w516 -> [w553]
                  tunnel: w515 -> [w552]
                  tunnel: w514 -> [w551]
                  tunnel: w513 -> [w550]
                  tunnel: [w549] -> w512
                  tunnel: [w548] -> w511
                  tunnel: w510 -> [w540]
                  i -> [w564]
                  n117 = Less Or Equal?(x=w564, y=w565) -> (x <= y?=w569:bool)
                  n118 = case shown="False" w569 {
                    tunnel: w568 -> [w581 w609]
                    tunnel: w564 -> [w590 w608]
                    tunnel: w567 -> [w589 w607]
                    tunnel: [w587 w605] -> w563
                    tunnel: w566 -> [w588 _]
                    tunnel: w565 -> [w583 _]
                    tunnel: w564 -> [w586 _]
                    frame False {
                      n119 = Multiply(x=w583, y=2) -> (x*y=w582:dbl)
                      n120 = Less Or Equal?(x=w586, y=w582) -> (x <= y?=w584:bool)
                      n121 = case shown="False" w584 {
                        tunnel: w590 -> [w597 w604]
                        tunnel: w589 -> [w595 w602]
                        tunnel: w588 -> [_ w600]
                        tunnel: [w593 w599] -> w587
                        tunnel: w583 -> [_ w598]
                        tunnel: w582 -> [w592 _]
                        tunnel: w581 -> [w591 _]
                        frame False {
                          n122 = Subtract(x=w597, y=w592) -> (x-y=w596:dbl)
                          n123 = Multiply(x=w595, y=w596) -> (x*y=w594:dbl)
                          n124 = Add(x=w591, y=w594) -> (x+y=w593:dbl)
                        }
                        frame True {
                          n125 = Subtract(x=w604, y=w598) -> (x-y=w603:dbl)
                          n126 = Multiply(x=w602, y=w603) -> (x*y=w601:dbl)
                          n127 = Subtract(x=w600, y=w601) -> (x-y=w599:dbl)
                        }
                      }
                    }
                    frame True {
                      n128 = Multiply(x=w607, y=w608) -> (x*y=w606:dbl)
                      n129 = Add(x=w609, y=w606) -> (x+y=w605:dbl)
                    }
                  }
                  n130 = Absolute Value(x=w563) -> (abs(x)=w562:dbl)
                  n131 = stacked-sequence {
                    tunnel: w571 -> [_ _ w710]
                    tunnel: w562 -> [w628 _ w648]
                    tunnel: w570 -> [_ _ w712]
                    tunnel: [_ _ w711] -> w558
                    tunnel: [_ _ w709] -> w543
                    tunnel: [_ _ w708] -> w547
                    tunnel: w561 -> [_ _ w707]
                    tunnel: [_ _ w706] -> w544
                    tunnel: [_ _ w705] -> w560
                    tunnel: w559 -> [_ _ w699]
                    tunnel: [_ _ w704] -> w557
                    tunnel: w556 -> [_ _ w700]
                    tunnel: [_ _ w703] -> w555
                    tunnel: w554 -> [_ _ w702]
                    tunnel: [_ _ w649] -> w545
                    tunnel: [_ _ w701] -> w546
                    tunnel: w553 -> [w627 _ _]
                    tunnel: w552 -> [w626 _ _]
                    tunnel: w551 -> [w623 _ _]
                    tunnel: w550 -> [_ w645 _]
                    tunnel: [w611 _ _] -> w549
                    tunnel: [w610 _ _] -> w548
                    tunnel: [_ _ w648] -> w541
                    frame #0 {
                      n132 = call "SetTemperature.vi"("Approach"="Sweep Temperature Approach", "Rate"="Sweep T  Rate (K/min)", "Temperature"=w628, "error in (no error)"=w626, "Instrument Ref In"=w627) -> ("error out"=w624:errorcluster, "Instrument Ref Out"=w625:refnum<k24>)  [unwired: 2 in, 1 out]
                      n133 = call "WaitFor.vi"("Delay"=w623, "Wait For Temperature"=TRUE ("WaitForTemperature"), "error in (no error)"=w624, "Instrument Ref In"=w625) -> ("error out"=w614:errorcluster, "Instrument Ref Out"=w613:refnum<k24>)  [unwired: 6 in]
                      n134 = for {
                        N: 20 -> [_]
                        shift-right: [w644] -> _
                        shift-left: TRUE -> [w642]
                        shift-right: [w639] -> w611
                        shift-left: w614 -> [w641]
                        tunnel: w613 -> [w638]
                        tunnel: [w636] -> w610
                        tunnel: [w633] -> w620
                        tunnel: [w632] -> w619
                        tunnel: [w634] -> w617 mode=indexing
                        tunnel: [w635] -> w618 mode=indexing
                        n135 = local write "Measuring T"(w642) -> ()
                        n136 = Not(x=w642) -> (.not. x?=w644:bool)
                        n137 = call "GetTemperature.vi"("error in (no error)"=w641, "Instrument Ref In"=w638) -> ("Temperature\nStatus"=w632:i32, "Temperature"=w635:dbl, "error out"=w640:errorcluster, "Instrument Ref Out"=w637:refnum<k24>)  [unwired: 3 in, 1 out]
                        n138 = Wait (ms)(milliseconds to wait=u32 200) -> ()  [unwired: 1 out]
                        n139 = call "GetField.vi"("error in (no error)"=w640, "Instrument Ref In"=w637) -> ("Field\nStatus"=w633:i32, "Field"=w634:dbl, "error out"=w639:errorcluster, "Instrument Ref Out"=w636:refnum<k24>)  [unwired: 3 in, 1 out]
                      }
                      "Field Status" <- w620
                      "Temperature Status" <- w619
                      n140 = call-poly <vilib>:"Mean.vi"("X"=w617) -> ("mean"=→"Fixed Field":dbl)  [unwired: 1 out]
                      n141 = call-poly <vilib>:"Mean.vi"("X"=w618) -> ("mean"=→"Measured Temperature":dbl)  [unwired: 1 out]
                      "Temperature Setting" <- w628
                      "Measuring T" <- FALSE
                    }
                    frame #1 {
                      n142 = Multiply(x=w645, y=1000) -> (x*y=w647:dbl)
                      n143 = Wait (ms)(milliseconds to wait=w647) -> ()  [unwired: 1 out]
                    }
                    frame #2 {
                      n144 = flat-sequence {
                        tunnel: w712 -> [w740]
                        tunnel: w710 -> [w731]
                        tunnel: w648 -> [w739]
                        tunnel: w707 -> [w738]
                        tunnel: w702 -> [w729]
                        tunnel: [w736] -> w698
                        tunnel: [w723] -> w696
                        tunnel: [w724] -> w694
                        tunnel: [w721] -> w692
                        tunnel: [w724] -> w690
                        tunnel: [w724] -> w688
                        tunnel: [w724] -> w686
                        tunnel: [w724] -> w684
                        tunnel: [w723] -> w682
                        tunnel: [w722] -> w680
                        tunnel: [w721] -> w678
                        tunnel: [w720] -> w676
                        tunnel: ["T Clear Plot B"] -> w674
                        tunnel: ["T Clear Plot A"] -> w672
                        tunnel: [w717] -> w670
                        tunnel: [w716] -> w668
                        tunnel: [w715] -> w666
                        tunnel: [w714] -> w664
                        tunnel: [w713] -> w662
                        tunnel: w698 -> [w762]
                        tunnel: [w762] -> w697
                        tunnel: w696 -> [w761]
                        tunnel: [w761] -> w695
                        tunnel: w694 -> [w760]
                        tunnel: [w760] -> w693
                        tunnel: w692 -> [w759]
                        tunnel: [w759] -> w691
                        tunnel: w690 -> [w758]
                        tunnel: [w758] -> w689
                        tunnel: w688 -> [w757]
                        tunnel: [w757] -> w687
                        tunnel: w686 -> [w756]
                        tunnel: [w756] -> w685
                        tunnel: w684 -> [w755]
                        tunnel: [w755] -> w683
                        tunnel: w682 -> [w754]
                        tunnel: [w754] -> w681
                        tunnel: w680 -> [w753]
                        tunnel: [w753] -> w679
                        tunnel: w678 -> [w752]
                        tunnel: [w752] -> w677
                        tunnel: w676 -> [w751]
                        tunnel: [w751] -> w675
                        tunnel: w674 -> [w750]
                        tunnel: [w750] -> w673
                        tunnel: w672 -> [w749]
                        tunnel: [w749] -> w671
                        tunnel: w670 -> [w748]
                        tunnel: [w748] -> w669
                        tunnel: w668 -> [w747]
                        tunnel: [w747] -> w667
                        tunnel: w666 -> [w746]
                        tunnel: [w746] -> w665
                        tunnel: w664 -> [w745]
                        tunnel: [w745] -> w663
                        tunnel: w662 -> [w744]
                        tunnel: [w744] -> w661
                        tunnel: w697 -> [w766]
                        tunnel: w695 -> [w800]
                        tunnel: w693 -> [w799]
                        tunnel: w691 -> [w798]
                        tunnel: w689 -> [w797]
                        tunnel: w687 -> [w795]
                        tunnel: w685 -> [w793]
                        tunnel: w683 -> [w791]
                        tunnel: w681 -> [w788]
                        tunnel: w679 -> [w787]
                        tunnel: w677 -> [w784]
                        tunnel: w675 -> [w783]
                        tunnel: w700 -> [w781]
                        tunnel: w673 -> [w780]
                        tunnel: w699 -> [w778]
                        tunnel: w671 -> [w777]
                        tunnel: w669 -> [w773]
                        tunnel: w667 -> [w772]
                        tunnel: w665 -> [w771]
                        tunnel: w663 -> [w768]
                        tunnel: w661 -> [w767]
                        tunnel: [w766] -> w660
                        tunnel: [w786] -> w659
                        tunnel: [w800] -> w658
                        tunnel: [w799] -> w657
                        tunnel: [w764] -> w656
                        tunnel: [w765] -> w655
                        tunnel: [w789] -> w654
                        tunnel: [w785] -> w653
                        tunnel: [w782] -> w652
                        tunnel: [w798] -> w651
                        tunnel: [w770] -> w650
                        tunnel: [w804] -> w701
                        tunnel: [w805] -> w649
                        tunnel: [w802] -> w703
                        tunnel: [w806] -> w704
                        tunnel: [w807] -> w705
                        tunnel: [w808] -> _
                        tunnel: [w809] -> w706
                        tunnel: [w810] -> w708
                        tunnel: [w811] -> w709
                        tunnel: [w801] -> w711
                        tunnel: [w812] -> _
                        tunnel: w660 -> [w812]
                        tunnel: w659 -> [w801]
                        tunnel: w658 -> [w811]
                        tunnel: w657 -> [w810]
                        tunnel: w656 -> [w809]
                        tunnel: w655 -> [w808]
                        tunnel: w654 -> [w807]
                        tunnel: w653 -> [w806]
                        tunnel: w652 -> [w802]
                        tunnel: w651 -> [w805]
                        tunnel: w650 -> [w804]
                        frame #0 {
                          w716 = u8 1 items=["Channel A", "Channel B"] ("Channel A/B for Parameter1")
                          w713 = u8 0 items=["Channel A", "Channel B"] ("Channel A/B for Parameter1")
                          n145 = Format Into String(0) -> (error out=w737:errorcluster)  [unwired: 3 in, 1 out]
                          n146 = Format Into String(0) -> (error out=w732:errorcluster)  [unwired: 3 in, 1 out]
                          n147 = call "OE1022D_Read 1 parameter_mean.vi"("错误输入（无错误）"=w737, "Parameter"="Parameter A", "Channel (0: A)"=w713, "VISA resource name"=w731) -> ("error out"=w714:errorcluster, "Measurement"=w726:dbl, "VISA resource name out"=w736:refnum<visa-resource-name>)  [unwired: 5 in]
                          n148 = call "OE1022D_Read 1 parameter_mean.vi"("Parameter 2"="Parameter B", "错误输入（无错误）"=w732, "Channel (0: A)"=w716, "VISA resource name"=w731) -> ("error out"=w717:errorcluster, "Measurement"=w725:dbl, "VISA resource name out"=w715:refnum<visa-resource-name>)  [unwired: 5 in]
                          n149 = Multiply(x=w726, y=1000.0) -> (x*y=w723:dbl)
                          "para1 Measurement (mV)" <- w723
                          n150 = Multiply(x=w725, y=1000000.0) -> (x*y=w721:dbl)
                          "para2 Measurement (uV)" <- w721
                          n151 = Build Array(w723) -> (w741:dbl[])
                          n152 = Build Array(w721) -> (w733:dbl[])
                          n153 = Select(t=w741, s="T Clear Plot A", f=w740) -> (s? t:f=w722:dbl[])
                          n154 = Select(t=w733, s="T Clear Plot B", f=w729) -> (s? t:f=w720:dbl[])
                          n155 = Build Array (concatenate)(w739, w738) -> (w724:dbl[])
                        }
                        frame #1 {
                          n156 = Wait (ms)(milliseconds to wait=u32 50) -> ()  [unwired: 1 out]
                        }
                        frame #2 {
                          n157 = Build Array (concatenate)(w788, w787) -> (w786:dbl[])
                          n158 = Build Array (concatenate)(w784, w783) -> (w782:dbl[])
                          n159 = Bundle(w793, w786) -> (→"RA-T":cluster{dbl[], dbl[]})  [unwired: 1 in]
                          n160 = Bundle(w795, w782) -> (→"Rh1B-T":cluster{dbl[], dbl[]})  [unwired: 1 in]
                          n161 = call "OE1022D_Read 1 parameter_mean.vi"("错误输入（无错误）"=w768, "Parameter"="Phase A", "Channel (0: A)"=w767, "VISA resource name"=w766) -> ("error out"=w765:errorcluster, "Measurement"=w764:dbl)  [unwired: 5 in, 1 out]
                          "phase A" <- w764
                          n162 = call "OE1022D_Read 1 parameter_mean.vi"("Parameter 2"="Phase B", "错误输入（无错误）"=w773, "Channel (0: A)"=w772, "VISA resource name"=w771) -> ("Measurement"=w770:dbl)  [unwired: 5 in, 2 out]
                          "phase B" <- w770
                          n163 = Build Array(w764) -> (w774:dbl[])
                          n164 = Build Array(w770) -> (w775:dbl[])
                          n165 = Select(t=w774, s=w777, f=w778) -> (s? t:f=w776:dbl[])
                          n166 = Select(t=w775, s=w780, f=w781) -> (s? t:f=w779:dbl[])
                          n167 = Build Array (concatenate)(w764, w776) -> (w789:dbl[])
                          n168 = Build Array (concatenate)(w770, w779) -> (w785:dbl[])
                          n169 = Bundle(w791, w789) -> (→"PhaseA-T":cluster{dbl[], dbl[]})  [unwired: 1 in]
                          n170 = Bundle(w797, w785) -> (→"Phaseh1-T":cluster{dbl[], dbl[]})  [unwired: 1 in]
                        }
                        frame #3 {
                          n171 = Wait (ms)(milliseconds to wait=u32 50) -> ()  [unwired: 1 out]
                        }
                      }
                    }
                  }
                  n172 = case shown="True" w540 {
                    tunnel: w543 -> [_ w575]
                    tunnel: w541 -> [_ w580]
                    tunnel: w542 -> [_ w578]
                    tunnel: w544 -> [_ w574]
                    tunnel: w545 -> [_ w573]
                    tunnel: w546 -> [_ w572]
                    frame False {
                    }
                    frame True {
                      n173 = Build Array(w580, w575, w574, w573, w572) -> (w577:dbl[])
                      n174 = call-poly <vilib>:"Write Delimited Spreadsheet.vi"("file path (dialog if empty)"=w578, "format (%.3f)"="%.10f", "1D data"=w577, "append to file? (new file:F)"=TRUE) -> ()  [unwired: 10 in, 2 out]
                    }
                  }
                }
              }
            }
          }
        }
      }
    }
    frame #2 {
      n175 = case shown="True" "Initialize" {
        tunnel: w815 -> [w816 w819]
        tunnel: w814 -> [w817 w818]
        frame False {
          n176 = Close Reference(reference=w817, error in (no error)=w816) -> ()  [unwired: 1 out]
        }
        frame True {
          w825 = 0 items=["Linear", "NoOvershoot", "Oscillate"] ("Approach")
          w826 = 0 items=["Persistent", "Driven"] ("Mode")
          w822 = 0 items=["FastSettle", "NoOvershoot"] ("Approach")
          n177 = call "SetTemperature.vi"("Approach"=w822, "Rate"=20.0, "Temperature"=120.0, "error in (no error)"=w819, "Instrument Ref In"=w818) -> ("error out"=w830:errorcluster, "Instrument Ref Out"=w829:refnum<k24>)  [unwired: 2 in, 1 out]
          n178 = call "SetField.vi"("Mode"=w826, "Approach"=w825, "Rate"=200.0, "Field"=0.0, "error in (no error)"=w830, "Instrument Ref In"=w829) -> ("error out"=w827:errorcluster, "Instrument Ref Out"=w828:refnum<k24>)  [unwired: 1 in, 1 out]
          n179 = Close Reference(reference=w828, error in (no error)=w827) -> ()  [unwired: 1 out]
        }
      }
    }
  }
  n180 = while {
    tunnel: w3 -> [w833]
    tunnel: w2 -> [w832]
    stop <- "?" stop-if-true
    n181 = for {
      N: 10 -> [_]
      shift-right: [w848] -> _
      shift-left: w832 -> [w850]
      tunnel: w833 -> [w847]
      tunnel: [w845] -> _
      tunnel: [w842] -> w839
      tunnel: [w841] -> w838
      tunnel: [w843] -> w836 mode=indexing
      tunnel: [w844] -> w837 mode=indexing
      n182 = call "GetTemperature.vi"("error in (no error)"=w850, "Instrument Ref In"=w847) -> ("Temperature\nStatus"=w841:i32, "Temperature"=w844:dbl, "error out"=w849:errorcluster, "Instrument Ref Out"=w846:refnum<k24>)  [unwired: 3 in, 1 out]
      n183 = Wait (ms)(milliseconds to wait=u32 200) -> ()  [unwired: 1 out]
      n184 = call "GetField.vi"("error in (no error)"=w849, "Instrument Ref In"=w846) -> ("Field\nStatus"=w842:i32, "Field"=w843:dbl, "error out"=w848:errorcluster, "Instrument Ref Out"=w845:refnum<k24>)  [unwired: 3 in, 1 out]
    }
    "Field Status" <- w839
    "Temperature Status" <- w838
    n185 = call-poly <vilib>:"Mean.vi"("X"=w836) -> ("mean"=→"Field":dbl)  [unwired: 1 out]
    n186 = call-poly <vilib>:"Mean.vi"("X"=w837) -> ("mean"=→"Temperature":dbl)  [unwired: 1 out]
  }
